vi "DoSpec.vi"() -> ()   [LabVIEW 2014]
uses:
  <userlib>/Nanonis Prog Interface V5/Nanonis Prog Interface.lvlib
panel:
  in  "ref setpoint":bool
  in  "start Bias (V)":sgl=-2.0 format="%_5p"
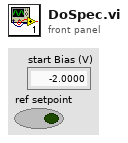
[diagram p1: front panel]
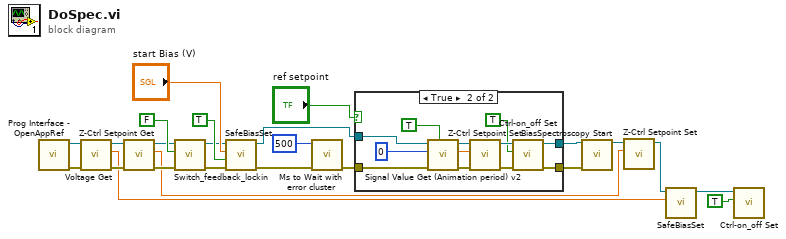
[diagram p0: block diagram]
diagram:
  n1 = call <userlib>:"Prog Interface - OpenAppRef.vi"() -> ("Error out"=w19:errorcluster, "Application reference"=w18:refnum<vi>)  [unwired: 6 in]
  n2 = call <userlib>:"Voltage Get.vi"("error in (no error)"=w19, "Application ref in"=w18) -> ("error out"=w16:errorcluster, "Bias (V)"=w11:sgl, "Application ref out"=w17:refnum<vi>)  [unwired: 7 in]
  n3 = call <userlib>:"Z-Ctrl Setpoint Get.vi"("error in (no error)"=w16, "Application ref in"=w17) -> ("error out"=w14:errorcluster, "Z Controller setpoint"=w10:sgl, "Application ref out"=w15:refnum<vi>)  [unwired: 6 in]
  n4 = call "Switch_feedback_lockin.vi"("error in (no error)"=w14, "Z Controller ON/OFF"=FALSE, "Application in"=w15) -> ("error out"=w4:errorcluster, "Application out"=w5:refnum<vi>)  [unwired: 7 in]
  n5 = call "SafeBiasSet.vi"("Application ref in"=w5, "Bias (V)"="start Bias (V)", "Ramp"=TRUE, "error in (no error)"=w4) -> ("Application ref out"=w6:refnum<vi>, "Error out"=w9:errorcluster)  [unwired: 5 in]
  n6 = call <userlib>:"Ms to Wait with error cluster.vi"("error in (no error)"=w9, "milliseconds to wait"=u32 500) -> ("error out"=w7:errorcluster)  [unwired: 4 in, 1 out]
  n7 = case shown="True" "ref setpoint" {
    tunnel: [w26 w35] -> w21
    tunnel: [w25 w34] -> w20
    tunnel: w7 -> [w25 w33]
    tunnel: w6 -> [w26 w31]
    frame False {
    }
    frame True {
      n8 = call <userlib>:"Signal Value Get (Animation period) v2.vi"("Wait for newest data (F=False)"=TRUE, "error in (no error)"=w33, "Signal index (0-79)"=i8 0, "Application ref in"=w31) -> ("error out"=w32:errorcluster, "Signal value"=w29:sgl, "Application ref out"=w30:refnum<vi>)  [unwired: 4 in]
      n9 = call <userlib>:"Z-Ctrl Setpoint Set.vi"("error in (no error)"=w32, "Z Controller setpoint"=w29, "Application ref in"=w30) -> ("error out"=w38:errorcluster, "Application ref out"=w37:refnum<vi>)  [unwired: 7 in]
      n10 = call <userlib>:"Ctrl-on_off Set.vi"("error in (no error)"=w38, "Z Controller ON/OFF"=TRUE, "Application ref in"=w37) -> ("error out"=w34:errorcluster, "Application ref out"=w35:refnum<vi>)  [unwired: 7 in]
    }
  }
  n11 = call <userlib>:"BiasSpectroscopy Start.vi"("Application ref in"=w21, "Error in (no error)"=w20) -> ("Application ref out"=w13:refnum<vi>)  [unwired: 9 in, 4 out]
  n12 = call <userlib>:"Z-Ctrl Setpoint Set.vi"("Z Controller setpoint"=w10, "Application ref in"=w13) -> ("Application ref out"=w12:refnum<vi>)  [unwired: 8 in, 1 out]
  n13 = call "SafeBiasSet.vi"("Application ref in"=w12, "Bias (V)"=w11) -> ("Application ref out"=w2:refnum<vi>)  [unwired: 7 in, 1 out]
  n14 = call <userlib>:"Ctrl-on_off Set.vi"("Z Controller ON/OFF"=TRUE, "Application ref in"=w2) -> ()  [unwired: 8 in, 2 out]
